vi "FPS_ColDet.vi"() -> (0 "Current FPS":i32)   [LabVIEW 2011]
uses:
  Enflo_Collision_Detection.dll
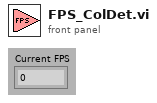
[diagram p1: front panel]
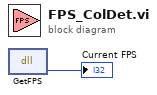
[diagram p0: block diagram]
diagram:
  n1 = dll-call lib="C:/Enflo_Software_SVN/EnFloSW/Anemometry/Anemometry Sub Vis/Collision_Detection/Enflo_Collision_Detection.dll" fn="GetFPS"() -> ("return type"=→"Current FPS":i32)  [unwired: 3 in, 2 out]
